vi "Command & Ack - Create Endpoints.vi"(8 "error in (no error)":errorcluster, 11 "SV B-M (Target) in":refnum<class "SV B-M (Target).lvclass">) -> (0 "error out":errorcluster, 3 "SV B-M (Target) out":refnum<class "SV B-M (Target).lvclass">)   [LabVIEW 2015, in "SV B-M (Target).lvclass"]
uses:
  SV B-M (Target).lvclass
  Type Defs/Message Cluster.ctl
  SV B-M (Target).lvclass/SV B-M (Target).ctl
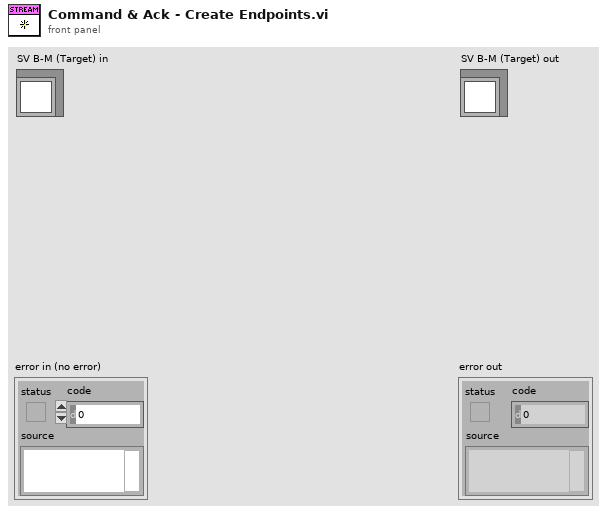
[diagram p1: front panel]
types:
  T1 = typedef "Message Cluster.ctl" = cluster{"Message":string, "Message Data":variant}
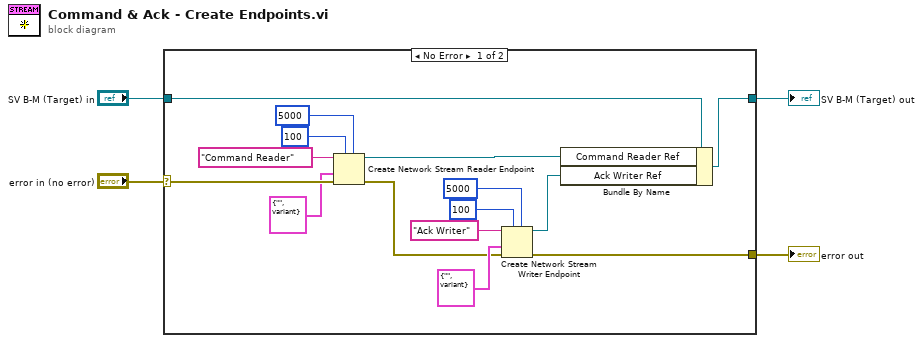
[diagram p0: block diagram]
diagram:
  n1 = case shown="No Error" "error in (no error)" {
    selector: "error in (no error)" -> [w18 w21]
    tunnel: [w5 w21] -> w4
    tunnel: [w7 w20] -> w2
    tunnel: "SV B-M (Target) in" -> [w8 w20]
    frame No Error {
      n2 = Create Network Stream Reader Endpoint(5:5000 ("timeout in ms (-1)"), 7:100 ("reader buffer size"), 8:w18, 9:T1 {"Message"="", "Message Data"=variant} ("Message Cluster"), 11:"Command Reader" ("reader name")) -> (0:w10:errorcluster, 3:w9:refnum<k21>)  [unwired: 2 in]
      n3 = Create Network Stream Writer Endpoint(5:5000 ("timeout in ms (-1)"), 7:100 ("reader buffer size"), 8:w10, 9:T1 {"Message"="", "Message Data"=variant} ("Message Cluster"), 11:"Ack Writer" ("reader name")) -> (0:w5:errorcluster, 3:w6:refnum<k21>)  [unwired: 2 in]
      n4 = Bundle By Name(cluster=w8, "Command Reader Ref"=w9, "Ack Writer Ref"=w6) -> (w7:refnum<class "SV B-M (Target).lvclass">)
    }
    frame Error {
    }
  }
  "error out" <- w4
  "SV B-M (Target) out" <- w2
